vi "Unbalance.vi"(0 "symmetrical components":T1, 9 "system info in":refnum<class "EP System Info.lvclass">, 11 "error in (no error)":errorcluster) -> (4 "unbalance":T1, 10 "system info out":refnum<class "EP System Info.lvclass">, 15 "error out":errorcluster)   [LabVIEW 2014, in "NI_EP_Power Quality.lvlib"]
doc: "Calculates the voltage and current unbalance for a three-phase electrical power system, according to IEC 61000-4-30:2008.\n\nThis VI supports measuring single-line and multiple-line systems."
uses:
  <vilib>/addons/Electrical Power/PQ/NI_EP_Power Quality.lvlib
  <vilib>/addons/Electrical Power/PQ/Common/Classes/System Info/EP System Info.lvclass
  <vilib>/addons/Electrical Power/Motor Monitoring/NI_EP_Motor Monitoring.lvlib
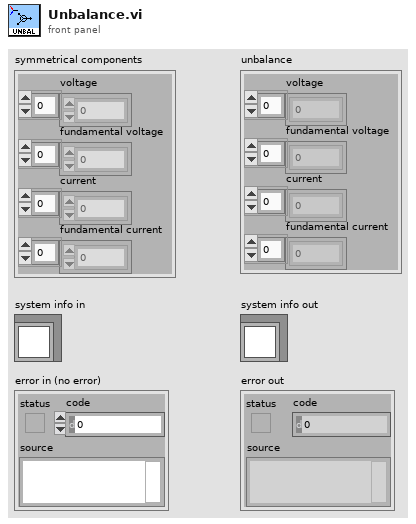
[diagram p1: front panel]
types:
  T1 = cluster{"voltage":dbl[], "fundamental voltage":dbl[], "current":dbl[], "fundamental current":dbl[]}
  T2 = cluster{"unbalance U":dbl[], "unbalance fund. U1":dbl[], "unbalance I":dbl[], "unbalance fund. I1":dbl[]}
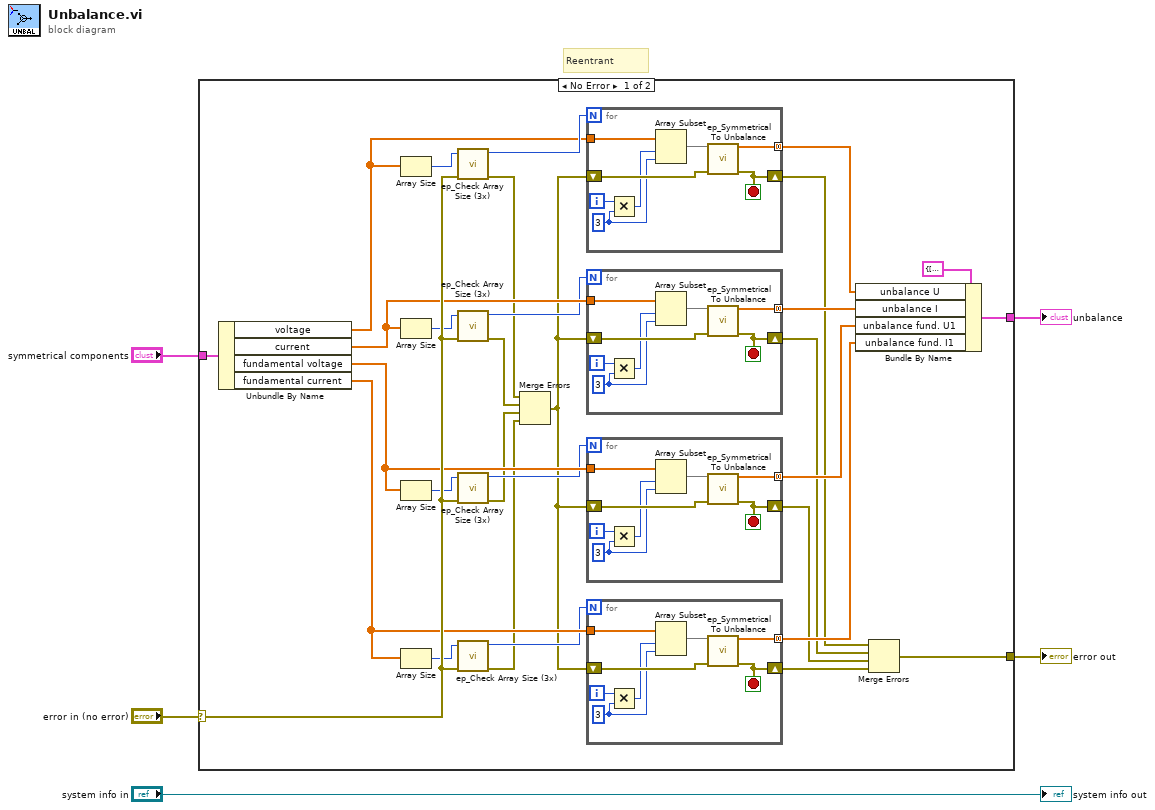
[diagram p0: block diagram]
diagram:
  # "Reentrant"
  n1 = case shown="No Error" "error in (no error)" {
    selector: "error in (no error)" -> [w31 w68]
    tunnel: "symmetrical components" -> [w35 _]
    tunnel: [w34 _] -> w2
    tunnel: [w15 w68] -> w1
    frame No Error {
      n2 = Unbundle By Name(w35) -> ("voltage"=w29:dbl[], "current"=w28:dbl[], "fundamental voltage"=w26:dbl[], "fundamental current"=w24:dbl[])
      n3 = Array Size(array=w29) -> (size(s)=w9:i32)
      n4 = Array Size(array=w28) -> (size(s)=w8:i32)
      n5 = Array Size(array=w26) -> (size(s)=w7:i32)
      n6 = Array Size(array=w24) -> (size(s)=w6:i32)
      n7 = call <vilib>:"ep_Check Array Size (3x).vi"("error in (no error)"=w31, "number of channels"=w9) -> ("error out"=w14:errorcluster, "number of 3 phases"=w30:i32)  [unwired: 8 in]
      n8 = call <vilib>:"ep_Check Array Size (3x).vi"("error in (no error)"=w31, "number of channels"=w8) -> ("error out"=w13:errorcluster, "number of 3 phases"=w27:i32)  [unwired: 8 in]
      n9 = call <vilib>:"ep_Check Array Size (3x).vi"("error in (no error)"=w31, "number of channels"=w7) -> ("error out"=w12:errorcluster, "number of 3 phases"=w25:i32)  [unwired: 8 in]
      n10 = call <vilib>:"ep_Check Array Size (3x).vi"("error in (no error)"=w31, "number of channels"=w6) -> ("error out"=w11:errorcluster, "number of 3 phases"=w23:i32)  [unwired: 8 in]
      n11 = Merge Errors(w14, w13, w12, w11) -> (w10:errorcluster)
      n12 = for {
        N: w30 -> [_]
        shift-right: [w65] -> w19
        shift-left: w10 -> [w66]
        tunnel: [w67] -> w32 mode=concatenating
        tunnel: w29 -> [w60]
        i -> [w62]
        stop <- w65 stop-if-true
        w64 = 3 ("x")
        n13 = Multiply(x=w62, y=w64) -> (x*y=w63:i32)
        n14 = Array Subset(array=w60, index=w63, length=w64) -> (w61:dbl[])
        n15 = call <vilib>:"ep_Symmetrical To Unbalance.vi"("symmetrical components"=w61, "error in (no error)"=w66) -> ("unbalance"=w67:dbl[], "error out"=w65:errorcluster)  [unwired: 12 in]
      }
      n16 = for {
        N: w27 -> [_]
        shift-right: [w57] -> w18
        shift-left: w10 -> [w58]
        tunnel: [w59] -> w22 mode=concatenating
        tunnel: w28 -> [w52]
        i -> [w54]
        stop <- w57 stop-if-true
        w56 = 3 ("x")
        n17 = Multiply(x=w54, y=w56) -> (x*y=w55:i32)
        n18 = Array Subset(array=w52, index=w55, length=w56) -> (w53:dbl[])
        n19 = call <vilib>:"ep_Symmetrical To Unbalance.vi"("symmetrical components"=w53, "error in (no error)"=w58) -> ("unbalance"=w59:dbl[], "error out"=w57:errorcluster)  [unwired: 12 in]
      }
      n20 = for {
        N: w25 -> [_]
        shift-right: [w49] -> w17
        shift-left: w10 -> [w50]
        tunnel: [w51] -> w21 mode=concatenating
        tunnel: w26 -> [w44]
        i -> [w46]
        stop <- w49 stop-if-true
        w48 = 3 ("x")
        n21 = Multiply(x=w46, y=w48) -> (x*y=w47:i32)
        n22 = Array Subset(array=w44, index=w47, length=w48) -> (w45:dbl[])
        n23 = call <vilib>:"ep_Symmetrical To Unbalance.vi"("symmetrical components"=w45, "error in (no error)"=w50) -> ("unbalance"=w51:dbl[], "error out"=w49:errorcluster)  [unwired: 12 in]
      }
      n24 = for {
        N: w23 -> [_]
        shift-right: [w41] -> w16
        shift-left: w10 -> [w42]
        tunnel: [w43] -> w20 mode=concatenating
        tunnel: w24 -> [w36]
        i -> [w38]
        stop <- w41 stop-if-true
        w40 = 3 ("x")
        n25 = Multiply(x=w38, y=w40) -> (x*y=w39:i32)
        n26 = Array Subset(array=w36, index=w39, length=w40) -> (w37:dbl[])
        n27 = call <vilib>:"ep_Symmetrical To Unbalance.vi"("symmetrical components"=w37, "error in (no error)"=w42) -> ("unbalance"=w43:dbl[], "error out"=w41:errorcluster)  [unwired: 12 in]
      }
      n28 = Bundle By Name(cluster=T2 {"unbalance U"=[], "unbalance fund. U1"=[], "unbalance I"=[], "unbalance fund. I1"=[]} ("unbalances"), "unbalance U"=w32, "unbalance I"=w22, "unbalance fund. U1"=w21, "unbalance fund. I1"=w20) -> (w34:T2)
      n29 = Merge Errors(w19, w18, w17, w16) -> (w15:errorcluster)
    }
    frame Error {
    }
  }
  "error out" <- w1
  "unbalance" <- w2
  "system info out" <- "system info in"
